vi "Get Default FPGA VI.vi"(9 "Target Project Path":path, 10 "Alias":string, 11 "LabVIEW Object in":refnum<class>) -> (3 "appended path":path)   [LabVIEW 2014, in "RIO Target.lvclass"]
uses:
  RIO Target.lvclass
  <vilib>/NI/Configuration Framework/class discovery singleton/class discovery singleton.lvlib
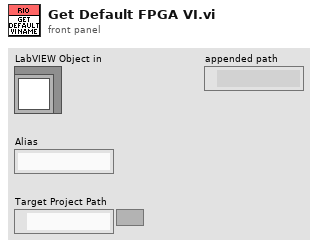
[diagram p1: front panel]
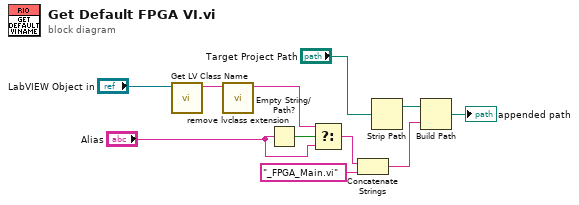
[diagram p0: block diagram]
diagram:
  n1 = call <vilib>:"Get LV Class Name.vi"("object"="LabVIEW Object in") -> ("class name"=w5:string)  [unwired: 9 in, 1 out]
  n2 = call <vilib>:"remove lvclass extension.vi"("class name in"=w5) -> ("class name out"=w6:string)  [unwired: 10 in]
  n3 = Empty String/Path?(string/path="Alias") -> (empty?=w3:bool)
  n4 = Select(t=w6, s=w3, f="Alias") -> (s? t:f=w8:string)
  n5 = Concatenate Strings(w8, "_FPGA_Main.vi" ("name or relative path")) -> (w9:string)
  n6 = Strip Path(path="Target Project Path") -> (stripped path=w2:path)  [unwired: 1 out]
  n7 = Build Path(base path=w2, name or relative path=w9) -> (appended path=→"appended path":path)
